vi "Create.vi"(8 "error in (no error)":errorcluster) -> (0 "error out":errorcluster, 3 "CLILogger out":refnum<class "CLILogger.lvclass">)   [LabVIEW 2020, in "GPackTools.lvlib" / "CLILogger.lvclass"]
uses:
  CLILogger.lvclass
  Log Entry.ctl
  CLILogger.lvclass/CLILogger.ctl
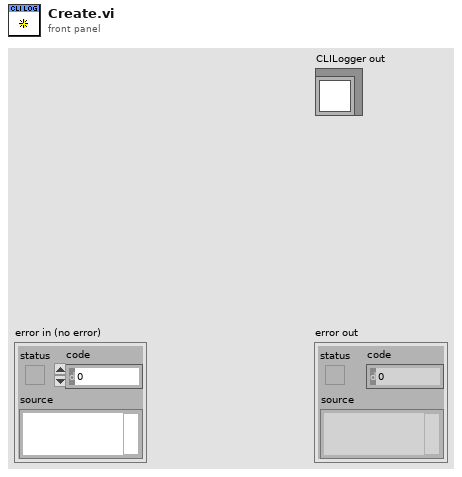
[diagram p1: front panel]
types:
  T1 = typedef "GPackTools.lvlib/CLILogger.lvclass/Log Entry.ctl" = cluster{"Time Stamp":timestamp, "Message":string}
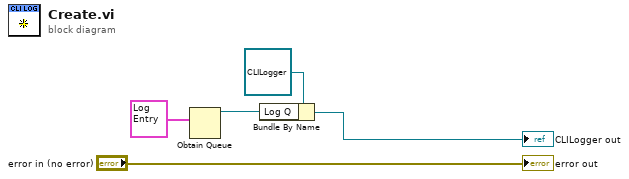
[diagram p0: block diagram]
diagram:
  n1 = Obtain Queue(element data type=T1 {"Time Stamp"=timestamp(0 s since 1904-01-01), "Message"=""} ("Log Entry")) -> (queue out=w1:refnum<queue>)  [unwired: 4 in, 2 out]
  n2 = Bundle By Name(cluster=refnum<class "CLILogger.lvclass"> refnum ("CLILogger in"), "Log Q"=w1) -> (→"CLILogger out":refnum<class "CLILogger.lvclass">)
  "error out" <- "error in (no error)"
